vi "_Python_Get_DT_and_AP_from_Histo.vi"(8 "error in (no error)":errorcluster, 11 "Histo path":path) -> (0 "error out":errorcluster, 1 "After Pulse":dbl format="%#_3f %", 2 "Dead Time":dbl format="%#_6p")   [LabVIEW 2018]
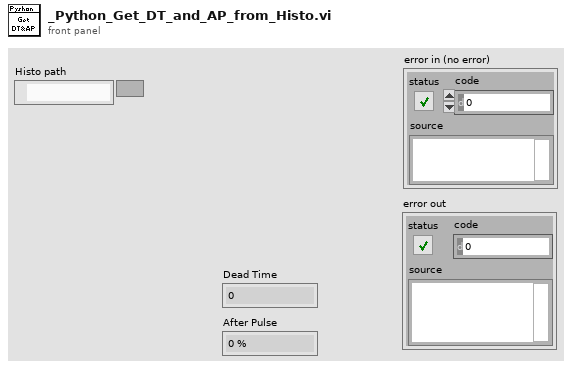
[diagram p1: front panel]
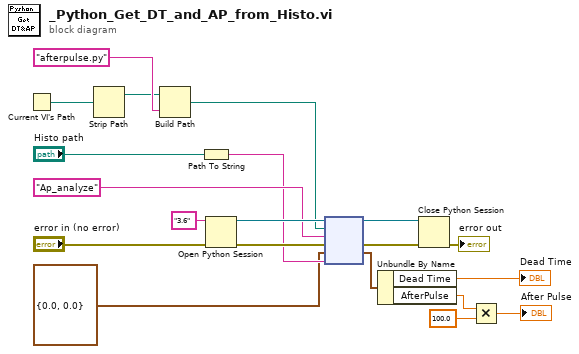
[diagram p0: block diagram]
diagram:
  n1 = Current VI's Path() -> (path=w13:path)
  n2 = Strip Path(path=w13) -> (stripped path=w10:path)  [unwired: 1 out]
  n3 = Build Path(base path=w10, name or relative path="afterpulse.py" ("function name")) -> (appended path=w11:path)
  n4 = Path To String(path="Histo path") -> (string=w9:string)
  n5 = Open Python Session(python version="3.6" ("Python version"), 3:"error in (no error)") -> (session out=w19:refnum<k35>, error out=w17:errorcluster)  [unwired: 1 in]
  n6 = node(w19, w11, "Ap_analyze" ("function name"), w17, cluster{"Dead Time":dbl, "AfterPulse":dbl} {"Dead Time"=0.0, "AfterPulse"=0.0}, w9) -> (w16:refnum<k35>, w15:errorcluster, w7:cluster{"Dead Time":dbl, "AfterPulse":dbl})  [unwired: 1 in, 2 out]
  n7 = Unbundle By Name(w7) -> ("Dead Time"=→"Dead Time":dbl, "AfterPulse"=w5:dbl)
  n8 = Close Python Session(session in=w16, error in=w15) -> (11:→"error out":errorcluster)
  n9 = Multiply(x=w5, y=100.0) -> (x*y=→"After Pulse":dbl)
